vi "ResetConditions.vi"(7 "data group":string, 8 "error in (no error)":errorcluster, 10 "map":T1, 11 "operating states in":variant) -> (0 "error out":errorcluster, 3 "operating states out":variant)   [LabVIEW 2017, in "OpState.lvlib"]
uses:
  <vilib>/addons/InsightCM/Devices/Shared/Common/OpState/OpState.lvlib
  <vilib>/addons/PointValueMap/controls/PointMap.ctl
  <vilib>/addons/InsightCM/Devices/Shared/Common/OpState/controls/TriggerOperatingState.ctl
  <vilib>/addons/InsightCM/MessageBus/Base/controls/KeyValuePair.ctl
  <vilib>/addons/InsightCM/Devices/Shared/Common/Trigger/controls/TriggerCondition.ctl
  <vilib>/addons/InsightCM/MessageBus/Base/controls/Condition.ctl
  <vilib>/addons/InsightCM/Devices/Shared/Common/Trigger/Trigger.lvlib
  <vilib>/addons/PointValueMap/PointValueMap.lvlib
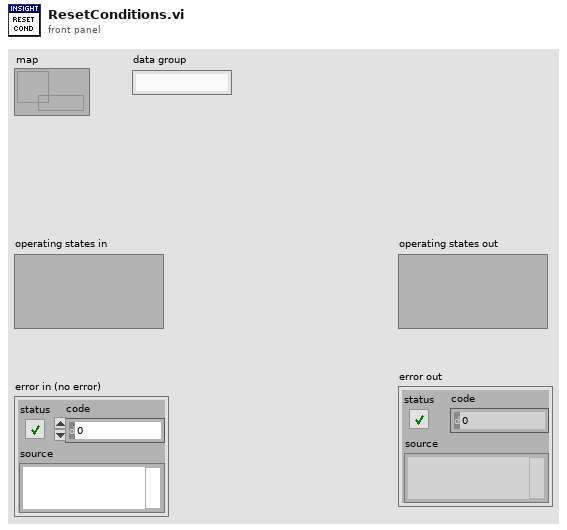
[diagram p1: front panel]
types:
  T1 = typedef "PointValueMap.lvlib/PointMap.ctl" = refnum<data-value>
  T2 = typedef "OpState.lvlib/TriggerOperatingState.ctl" = cluster{"Id":string, "Name":string, "Properties":T3[], "EnterExpression":string, "EnterConditions":T4[], "ExitExpression":string, "ExitConditions":T4[]}
  T3 = typedef "KeyValuePair.ctl" = cluster{"Key":string, "Value":string}
  T4 = typedef "Trigger.lvlib/TriggerCondition.ctl" = cluster{"Condition":T5, "LatchValue":string, "LatchTime":timestamp}
  T5 = typedef "Condition.ctl" = cluster{"Source":string, "Type":string, "Operator":string, "CompareTo":string, "DwellSeconds":dbl}
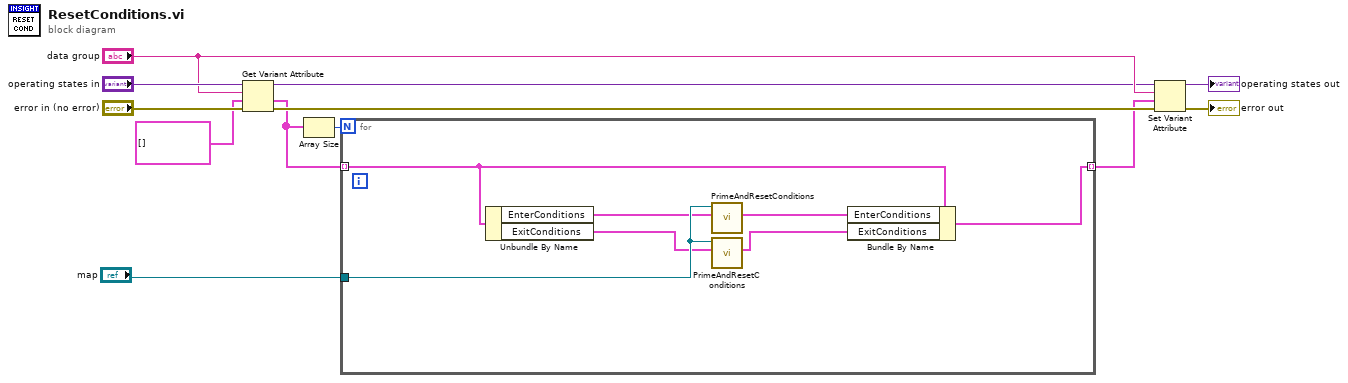
[diagram p0: block diagram]
diagram:
  n1 = Get Variant Attribute(Variant="operating states in", name="data group", default value (empty Variant)=T2[] [] ("OperatingStates"), error in="error in (no error)") -> (duplicate Variant=w5:variant, value=w2:T2[], error out=w9:errorcluster)  [unwired: 1 out]
  n2 = Array Size(array=w2) -> (size(s)=w1:i32)
  n3 = for {
    N: w1 -> [_]
    tunnel: w2 -> [w14] mode=indexing
    tunnel: [w13] -> w7 mode=indexing
    tunnel: "map" -> [w19]
    n4 = Unbundle By Name(w14) -> ("EnterConditions"=w18:T4[], "ExitConditions"=w17:T4[])
    n5 = call <vilib>:"PrimeAndResetConditions.vi"("conditions in"=w18, "SnapshotMap"=w19) -> ("conditions out"=w16:T4[])  [unwired: 8 in, 1 out]
    n6 = call <vilib>:"PrimeAndResetConditions.vi"("conditions in"=w17, "SnapshotMap"=w19) -> ("conditions out"=w15:T4[])  [unwired: 8 in, 1 out]
    n7 = Bundle By Name(cluster=w14, "EnterConditions"=w16, "ExitConditions"=w15) -> (w13:T2)
  }
  n8 = Set Variant Attribute(Variant=w5, name="data group", value=w7, error in=w9) -> (Variant out=→"operating states out":variant, error out=→"error out":errorcluster)  [unwired: 1 out]
